vi "Read_LegProperties.vi"(8 "error in (no error)":errorcluster, 11 "CAlex2 in":refnum<class "CAlex2.lvclass">) -> (0 "error out":errorcluster, 2 "LegProperties":T1, 3 "CAlex2 out":refnum<class "CAlex2.lvclass">)   [LabVIEW 2016, in "CAlex2.lvclass"]
uses:
  CAlex2.lvclass
  TypeDef/LowerBodyDim.ctl
  CAlex2.lvclass/CAlex2.ctl
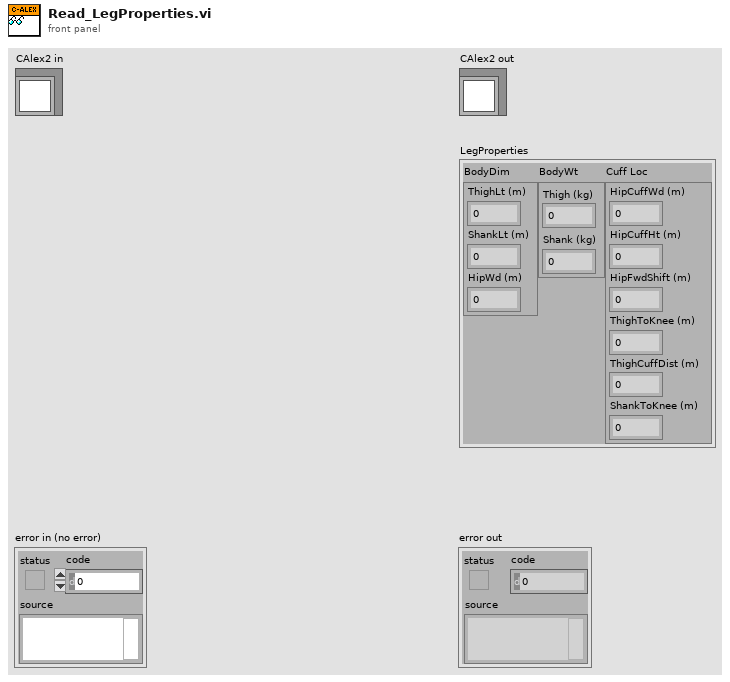
[diagram p1: front panel]
types:
  T1 = typedef "CAlex2.lvclass/LowerBodyDim.ctl" = cluster{"BodyDim":cluster{"ThighLt (m)":dbl, "ShankLt (m)":dbl, "HipWd (m)":dbl}, "BodyWt":cluster{"Thigh (kg)":dbl, "Shank (kg)":dbl}, "Cuff Loc":cluster{"HipCuffWd (m)":dbl, "HipCuffHt (m)":dbl, "HipFwdShift (m)":dbl, "ThighToKnee (m)":dbl, "ThighCuffDist (m)":dbl, "ShankToKnee (m)":dbl}}
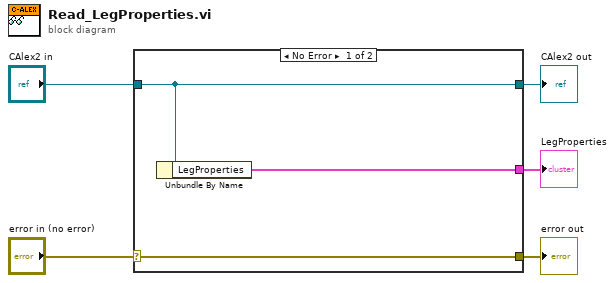
[diagram p0: block diagram]
diagram:
  n1 = case shown="No Error" "error in (no error)" {
    selector: "error in (no error)" -> [w8 w9]
    tunnel: [w8 w9] -> w4
    tunnel: [w7 w10] -> w2
    tunnel: "CAlex2 in" -> [w7 w10]
    tunnel: [w6 _] -> w1
    frame No Error {
      n2 = Unbundle By Name(w7) -> ("LegProperties"=w6:T1)
    }
    frame Error {
    }
  }
  "error out" <- w4
  "CAlex2 out" <- w2
  "LegProperties" <- w1
